vi "VI Tree.vi"   [LabVIEW 2011, in "Template - Function Generator.lvlib"]
doc: "This is the instrument driver for the <INSTRUMENT NAME>. The VI Tree displays all the user-callable VIs of the instrument driver in an organized table."
uses:
  <instrlib>/_Template - Function Generator/Template - Function Generator.lvlib
  <instrlib>/_Template - Function Generator/Public/Configure/Configure Modulation (Amplitude).vi
panel:
  # "(c) 2007 <Enter Company Name Here>.  ALL RIGHTS RESERVED."
  # "SEE DIAGRAM\nFOR VI TREE."
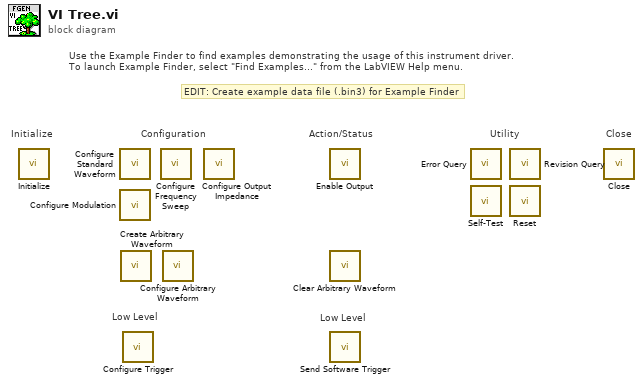
[diagram p0: block diagram]
diagram:
  # "EDIT: Create example data file (.bin3) for Example Finder"
  # "Low Level"
  # "Low Level"
  # "Use the Example Finder to find examples demonstrating the usage of this instrument driver.\nTo launch Example Finder, select \"Find Examples...\" from the LabVIEW Help menu."
  # "Configuration"
  # "Utility"
  # "Action/Status"
  # "Close"
  # "Initialize"
  n1 = call <instrlib>:"Initialize.vi"() -> ()  [unwired: 10 in, 2 out]
  n2 = call <instrlib>:"Configure Standard Waveform.vi"() -> ()  [unwired: 10 in, 2 out]
  n3 = call-poly <instrlib>:"Configure Modulation.vi"() -> ()  [unwired: 10 in, 2 out]
  n4 = call <instrlib>:"Create Arbitrary Waveform.vi"() -> ()  [unwired: 10 in, 2 out]
  n5 = call <instrlib>:"Configure Trigger.vi"() -> ()  [unwired: 10 in, 2 out]
  n6 = call <instrlib>:"Configure Frequency Sweep.vi"() -> ()  [unwired: 10 in, 2 out]
  n7 = call <instrlib>:"Configure Arbitrary Waveform.vi"() -> ()  [unwired: 10 in, 2 out]
  n8 = call <instrlib>:"Configure Output Impedance.vi"() -> ()  [unwired: 10 in, 2 out]
  n9 = call <instrlib>:"Enable Output.vi"() -> ()  [unwired: 10 in, 2 out]
  n10 = call <instrlib>:"Clear Arbitrary Waveform.vi"() -> ()  [unwired: 10 in, 2 out]
  n11 = call <instrlib>:"Send Software Trigger.vi"() -> ()  [unwired: 10 in, 2 out]
  n12 = call <instrlib>:"Error Query.vi"() -> ()  [unwired: 8 in, 4 out]
  n13 = call <instrlib>:"Self-Test.vi"() -> ()  [unwired: 8 in, 4 out]
  n14 = call <instrlib>:"Revision Query.vi"() -> ()  [unwired: 8 in, 4 out]
  n15 = call <instrlib>:"Reset.vi"() -> ()  [unwired: 10 in, 2 out]
  n16 = call <instrlib>:"Close.vi"() -> ()  [unwired: 11 in, 1 out]
